vi "SSL_Write.vi"(8 "error in (no error)":errorcluster, 10 "data in":u8[](array[numeric]) format="%x", 11 "SSL_Connection":T1) -> (0 "error out":errorcluster, 3 "SSL_Connection":T1)   [LabVIEW 2016, in "AWS_IoT.lvlib"]
doc: "MIT License\n\nCopyright (c) 2016 Indie-Energy\n\nPermission is hereby granted, free of charge, to any person obtaining a copy\nof this software and associated documentation files (the \"Software\"), to deal\nin the Software without restriction, including without limitation the rights\nto use, copy, modify, merge, publish, distribute, sublicense, and/or sell\ncopies of the Software, and to permit persons to whom the Software is\nfurnished to do so, subject to the following conditions:\n\nThe above copyright notice and this permission notice shall be included in all\ncopies or substantial portions of the Software.\n\nTHE SOFTWARE IS PROVIDED \"AS IS\", WITHOUT WARRANTY OF ANY KIND, EXPRESS OR\nIMPLIED, INCLUDING BUT NOT LIMITED TO THE WARRANTIES OF MERCHANTABILITY,\nFITNESS FOR A PARTICULAR PURPOSE AND NONINFRINGEMENT. IN NO EVENT SHALL THE\nAUTHORS OR COPYRIGHT HOLDERS BE LIABLE FOR ANY CLAIM, DAMAGES OR OTHER\nLIABILITY, WHETHER IN AN ACTION OF CONTRACT, TORT OR OTHERWISE, ARISING FROM,\nOUT OF OR IN CONNECTION WITH THE SOFTWARE OR THE USE OR OTHER DEALINGS IN THE\nSOFTWARE."
uses:
  AWS_IoT.lvlib
  Controls/SSL_Connection.ctl
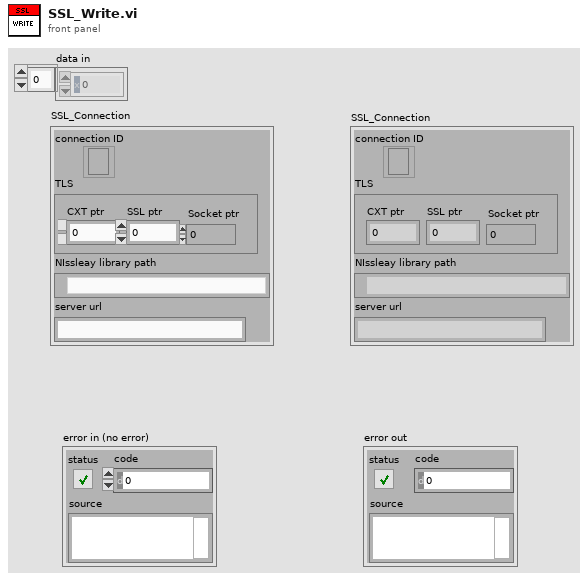
[diagram p1: front panel]
types:
  T1 = typedef "AWS_IoT.lvlib/SSL_Connection.ctl" = cluster{"connection ID":refnum<k5>, "TLS":cluster{"CXT ptr":i32, "SSL ptr":i32, "Socket ptr":i32}, "NIssleay library path":path, "server url":string}
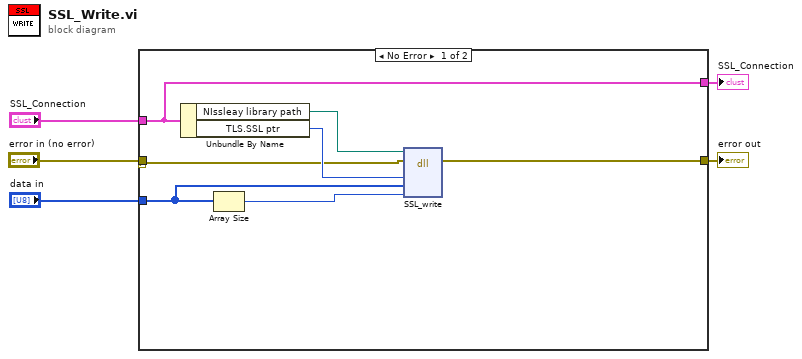
[diagram p0: block diagram]
diagram:
  n1 = case shown="No Error" "error in (no error)" {
    selector: "error in (no error)" -> [w6 w13]
    tunnel: "SSL_Connection" -> [w7 w14]
    tunnel: "data in" -> [w10 _]
    tunnel: [w6 w13] -> _
    tunnel: [w8 w13] -> w3
    tunnel: [w7 w14] -> w2
    frame No Error {
      n2 = Unbundle By Name(w7) -> ("NIssleay library path"=w12:path, "TLS.SSL ptr"=w11:i32)
      n3 = Array Size(array=w10) -> (size(s)=w9:i32)
      n4 = dll-call lib="NIssleay32.*" fn="SSL_write"(path in=w12, error in=w6, "SSL"=w11, "stringBuf"=w10, "stringLen"=w9) -> (error out=w8:errorcluster)  [unwired: 5 in, 1 out]
    }
    frame Error {
    }
  }
  "error out" <- w3
  "SSL_Connection" <- w2
